vi "_GenerateStateMap.vi"(8 "error in (no error)":errorcluster, 11 "Rules":T1[](array[typedef])) -> (0 "error out":errorcluster, 2 "StateNames":string[](array[string]), 3 "RulesMap":variant[](array[variant]))   [LabVIEW 2017, in "UIStateExpression.lvlib"]
uses:
  UIStateExpression/UIStateExpression.lvlib
  Typedef/RefMgr-Logic-State.ctl
  Typedef/RefMgr-StateChangeType.ctl
  f57af8ee-580f-41b0-a8dd-5ec74dddaa51.vi
  <userlib>/_OpenG.lib/array/array.llb/Remove Duplicates from 1D Array (String)__ogtk.vi
  <userlib>/_OpenG.lib/array/array.llb/Search 1D Array (String)__ogtk.vi
  TagDB RefManager.lvlib
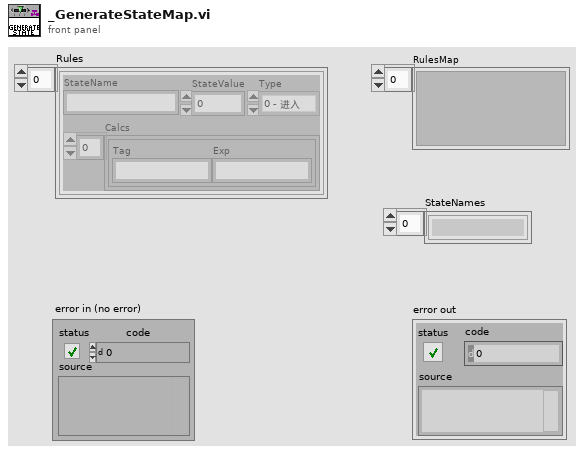
[diagram p1: front panel]
types:
  T1 = typedef "TagDB RefManager.lvlib/RefMgr-Logic-State.ctl" = cluster{"StateName":string, "StateValue":i32, "Type":T2, "Calcs":cluster{"Tag":string, "Exp":string}[]}
  T2 = typedef "TagDB RefManager.lvlib/RefMgr-StateChangeType.ctl" = enum16{"0 - 进入", "1 - 等于", "2 - 退出"}
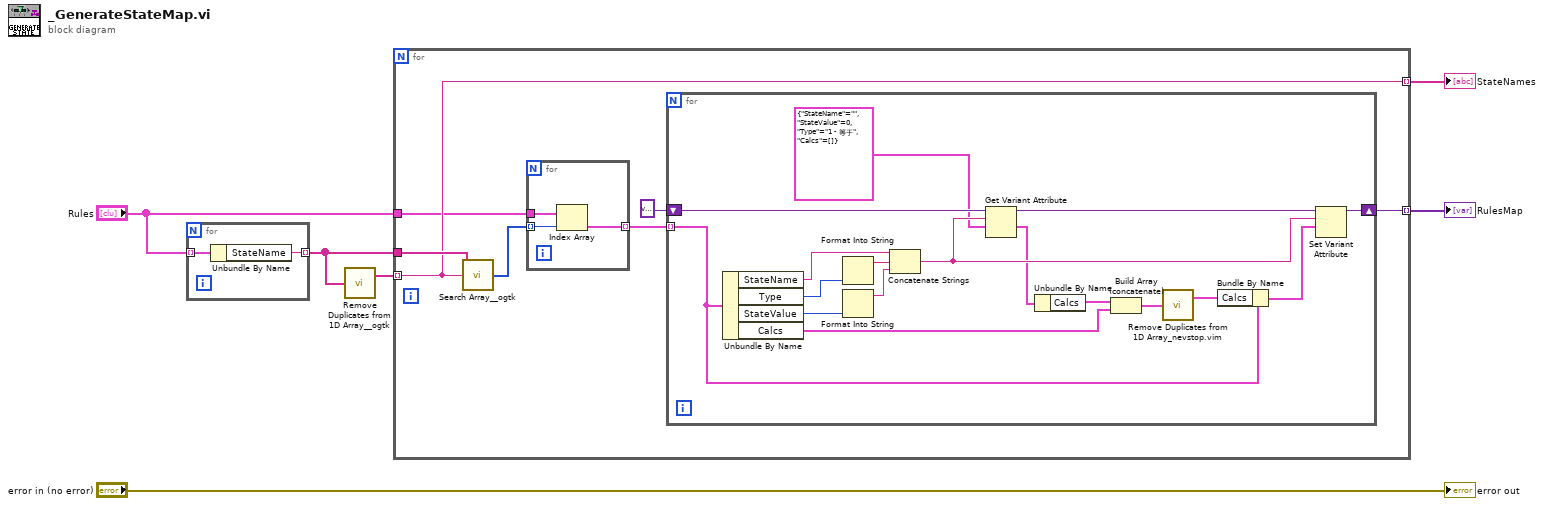
[diagram p0: block diagram]
diagram:
  n1 = for {
    tunnel: "Rules" -> [w8] mode=indexing
    tunnel: [w7] -> w3 mode=indexing
    n2 = Unbundle By Name(w8) -> ("StateName"=w7:string)
  }
  n3 = call-poly <userlib>:"Remove Duplicates from 1D Array__ogtk.vi"("Input Array"=w3) -> ("Output Array"=w2:string[])  [unwired: 1 out]
  n4 = for {
    tunnel: w2 -> [w13] mode=indexing
    tunnel: w3 -> [w15]
    tunnel: "Rules" -> [w11]
    tunnel: [w12] -> w6 mode=indexing
    tunnel: [w13] -> w5 mode=indexing
    n5 = call-poly <userlib>:"Search Array__ogtk.vi"("Array"=w15, "Element Data"=w13) -> ("Indices of Elements"=w10:i32[])  [unwired: 7 in]
    n6 = for {
      tunnel: w10 -> [w18] mode=indexing
      tunnel: w11 -> [w17]
      tunnel: [w16] -> w9 mode=indexing
      n7 = Index Array(array=w17, index=w18) -> (element=w16:T1)
    }
    n8 = for {
      tunnel: w9 -> [w22] mode=indexing
      shift-right: [w35] -> w12
      shift-left: variant ("variant") -> [w29]
      n9 = Unbundle By Name(w22) -> ("StateName"=w34:string, "Type"=w33:T2, "StateValue"=w31:i32, "Calcs"=w24:cluster{"Tag":string, "Exp":string}[])
      n10 = Format Into String(w33) -> (resulting string=w32:string)  [unwired: 3 in, 1 out]
      n11 = Format Into String(w31) -> (resulting string=w30:string)  [unwired: 3 in, 1 out]
      n12 = Concatenate Strings(w34, w32, w30) -> (w27:string)
      n13 = Get Variant Attribute(Variant=w29, name=w27, default value (empty Variant)=T1 {"StateName"="", "StateValue"=0, "Type"=enum."1 - 等于", "Calcs"=[]} ("Cluster")) -> (duplicate Variant=w28:variant, value=w26:T1)  [unwired: 1 in, 2 out]
      n14 = Unbundle By Name(w26) -> ("Calcs"=w25:cluster{"Tag":string, "Exp":string}[])
      n15 = Build Array (concatenate)(w25, w24) -> (w19:cluster{"Tag":string, "Exp":string}[])
      n16 = call "Remove Duplicates from 1D Array_nevstop.vim"("Input Array"=w19) -> ("Output Array"=w21:cluster{"Tag":string, "Exp":string}[])  [unwired: 1 out]
      n17 = Bundle By Name(cluster=w22, "Calcs"=w21) -> (w20:T1)
      n18 = Set Variant Attribute(Variant=w28, name=w27, value=w20) -> (Variant out=w35:variant)  [unwired: 1 in, 2 out]
    }
  }
  "RulesMap" <- w6
  "StateNames" <- w5
  "error out" <- "error in (no error)"
